vi "AMC Three Button Dialog Example.vi"() -> ()   [LabVIEW 2017]
panel:
  out "Waveform Chart":dbl(graph)
  in  "stop":bool
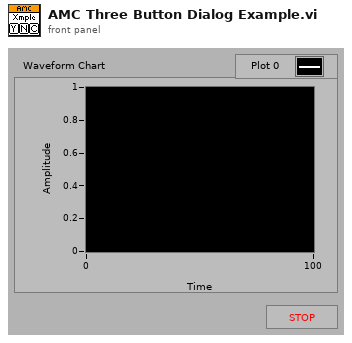
[diagram p1: front panel]
types:
  T1 = enum16{"Left Button", "Center Button", "Right Button", "Window Close"}
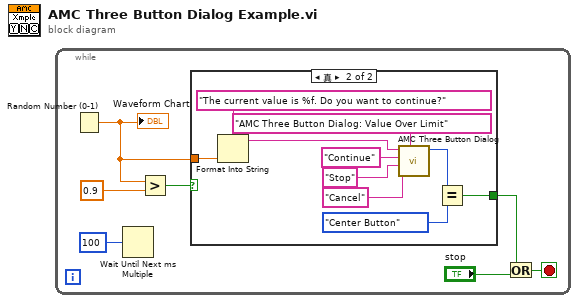
[diagram p0: block diagram]
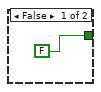
[diagram p2: hidden frame]
diagram:
  n1 = while {
    stop <- w1 stop-if-true
    n2 = Random Number (0-1)() -> (number: 0 to 1=w4:dbl)
    "Waveform Chart" <- w4
    n3 = Wait Until Next ms Multiple(millisecond multiple=u32 100) -> ()  [unwired: 1 out]
    n4 = Greater?(x=w4, y=0.9) -> (0:w5:bool)
    n5 = case shown="真" w5 {
      tunnel: w4 -> [_ w18]
      tunnel: [FALSE w10] -> w3
      frame False {
      }
      frame True {
        n6 = Format Into String(format string="The current value is %f. Do you want to continue?", w18) -> (resulting string=w17:string)  [unwired: 2 in, 1 out]
        n7 = call "AMC Three Button Dialog.vi"("Window Title (\"\")"="AMC Three Button Dialog: Value Over Limit" ("Dialog Title"), "Right Button Text (\"Cancel\")"="Cancel" ("Right Button Text"), "Center Button Text (\"No\")"="Stop" ("Center Button Text"), "Left Button Text (\"Yes\")"="Continue" ("Left Button Text"), "message"=w17) -> ("Which Button?"=w12:T1)  [unwired: 6 out]
        n8 = Equal?(x=w12, y=T1."Center Button") -> (x = y?=w10:bool)
      }
    }
    n9 = Or(x=w3, y="stop") -> (x .or. y?=w1:bool)
  }
